vi "usb_get_data.vi"(7 "byVdCmdHeaderLen":u16, 8 "error in":errorcluster, 9 "I2C_VD_BUFFER_RW":u16, 10 "I2C_SLAVE_ID":u8, 11 "data":u8[](array[numeric])) -> (0 "error out":errorcluster, 2 "data out":u8[](array[numeric]), 3 "return":i32)   [LabVIEW 2016]
uses:
  Global variable.vi
panel:
  in  "usb_ctl_info_t":T1
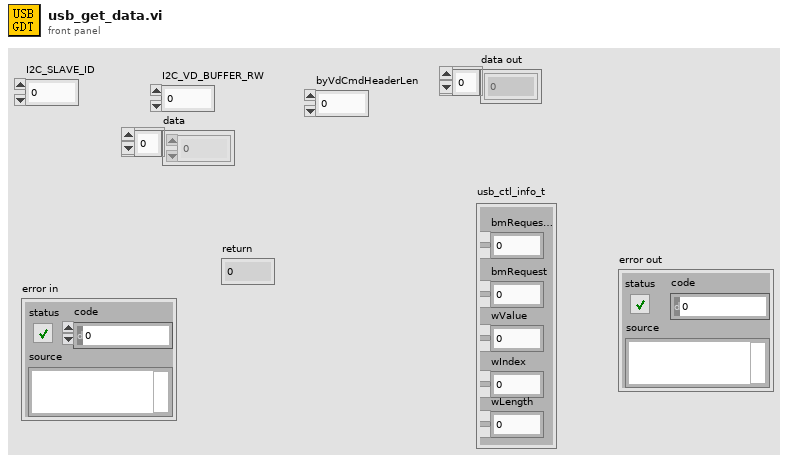
[diagram p1: front panel]
types:
  T1 = cluster{"bmRequestType":u8, "bmRequest":u8, "wValue":u16, "wIndex":u16, "wLength":u16}
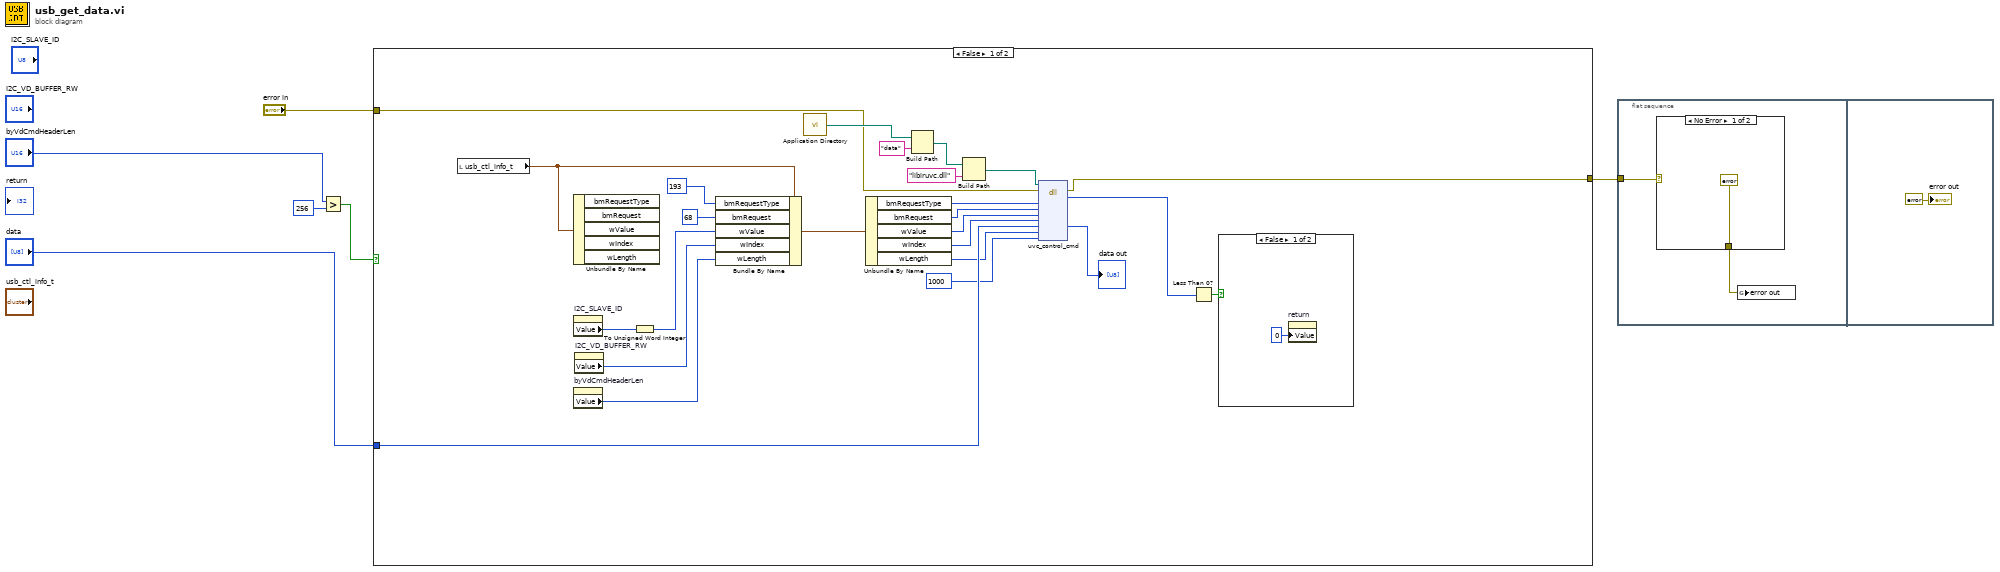
[diagram p0: block diagram]
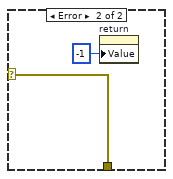
[diagram p2: hidden frame]
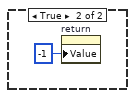
[diagram p3: hidden frame]
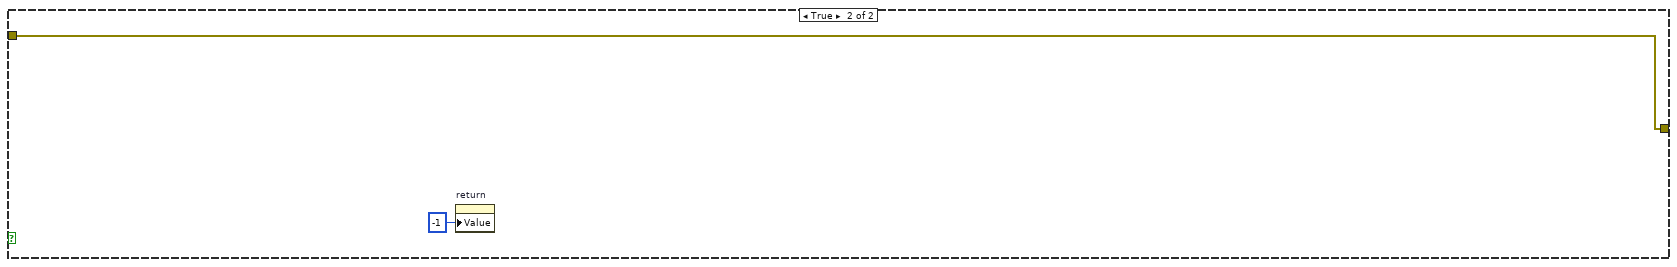
[diagram p4: hidden frame]
diagram:
  n1 = Greater?(x="byVdCmdHeaderLen", y=u16 256) -> (0:w4:bool)
  n2 = case shown="False" w4 {
    tunnel: "data" -> [w16 _]
    tunnel: "error in" -> [w10 w34]
    tunnel: [w9 w34] -> w1
    frame False {
      n3 = local read "usb_ctl_info_t"() -> (w31:T1)
      n4 = Unbundle By Name(w31) -> ()  [unwired: 5 out]
      n5 = property on="I2C_SLAVE_ID" class="DigNum (strict)"() -> ("Value"=w28:u8)  [unwired: 2 in, 2 out]
      n6 = property on="byVdCmdHeaderLen" class="DigNum (strict)"() -> ("Value"=w26:u16)  [unwired: 2 in, 2 out]
      n7 = property on="I2C_VD_BUFFER_RW" class="DigNum (strict)"() -> ("Value"=w27:u16)  [unwired: 2 in, 2 out]
      n8 = To Unsigned Word Integer(number=w28) -> (unsigned 16bit integer=w13:u16)
      n9 = Bundle By Name(cluster=w31, "bmRequestType"=u8 193, "bmRequest"=u8 68, "wValue"=w13, "wIndex"=w27, "wLength"=w26) -> (w21:T1)
      n10 = call <vilib>:"Application Directory.vi"() -> ("Application Directory"=w11:path)
      n11 = Unbundle By Name(w21) -> ("bmRequestType"=w20:u8, "bmRequest"=w19:u8, "wValue"=w18:u16, "wIndex"=w17:u16, "wLength"=w15:u16)
      n12 = Build Path(base path=w11, name or relative path="data") -> (appended path=w23:path)
      n13 = Build Path(base path=w23, name or relative path="libiruvc.dll") -> (appended path=w22:path)
      n14 = dll-call lib="PTH29abs EMyFolderISP上位机开发datalibiruvc.dll" fn="uvc_control_cmd"(path in=w22, error in=w10, "bmRequestType"=w20, "bRequest"=w19, "wValue"=w18, "wIndex"=w17, "data"=w16, "wLength"=w15, "timeout"=u32 1000) -> (error out=w9:errorcluster, "return type"=w7:i32, "data"=→"data out":u8[])  [unwired: 7 in, 1 out]
      n15 = Less Than 0?(x=w7) -> (x < 0?=w8:bool)
      n16 = case shown="False" w8 {
        frame False {
          n17 = property on="return" class="DigNum (strict)"("Value"=0 ("return")) -> ()  [unwired: 2 in, 2 out]
        }
        frame True {
          n18 = property on="return" class="DigNum (strict)"("Value"=-1 ("return")) -> ()  [unwired: 2 in, 2 out]
        }
      }
    }
    frame True {
      n19 = property on="return" class="DigNum (strict)"("Value"=-1 ("return")) -> ()  [unwired: 2 in, 2 out]
    }
  }
  n20 = flat-sequence {
    tunnel: w1 -> [w37]
    frame #0 {
      n21 = case shown="No Error" w37 {
        selector: w37 -> [_ w39]
        tunnel: [errorcluster {"status"=FALSE, "code"=0, "source"="successful"} ("error IO") w39] -> w36
        frame No Error {
        }
        frame Error {
          n22 = property on="return" class="DigNum (strict)"("Value"=-1 ("return")) -> ()  [unwired: 2 in, 2 out]
        }
      }
      n23 = global write "Global variable.vi" "error out"(w36) -> ()
    }
    frame #1 {
      "error out" <- errorcluster {"status"=FALSE, "code"=0, "source"=""} ("error out")
    }
  }
